vi "CloseTrig.vi"(8 "error in (no error)":errorcluster, 10 "TrigName":string, 11 "PXI_MultiTrig in":refnum<class "PXI_MultiTrig.lvclass">) -> (0 "error out":errorcluster, 3 "PXI_MultiTrig out":refnum<class "PXI_MultiTrig.lvclass">)   [LabVIEW 2018, in "SyncPlugins.lvlib" / "PXI_MultiTrig.lvclass"]
uses:
  PXI_MultiTrig.lvclass
  PXI_MultiTrig.lvclass/PXI_MultiTrig.ctl
  Accessors/Write TimingSession.vi
  Accessors/Write Triggers.vi
  Accessors/Read TimingSession.vi
  Accessors/Read RefClkSession.vi
  Accessors/Read Triggers.vi
  <vilib>/Utility/error.llb/Error Cluster From Error Code.vi
  <vilib>/ErrorRing/Error Ring.xnode
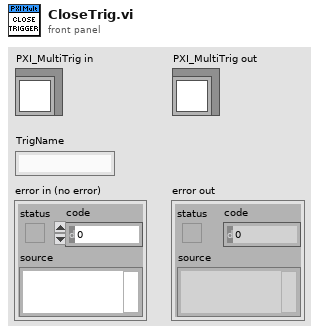
[diagram p1: front panel]
types:
  T1 = typedef "SyncPlugins.lvlib/PXI_MultiTrig.lvclass/clTrigger.ctl" = cluster{"Name":string, "DestTerm":string, "SrcTerm":string, "SyncClk":string, "Edge":i32, "Invert?":i32, "Initiated":bool, "Type":string, "TrigTime":bool}
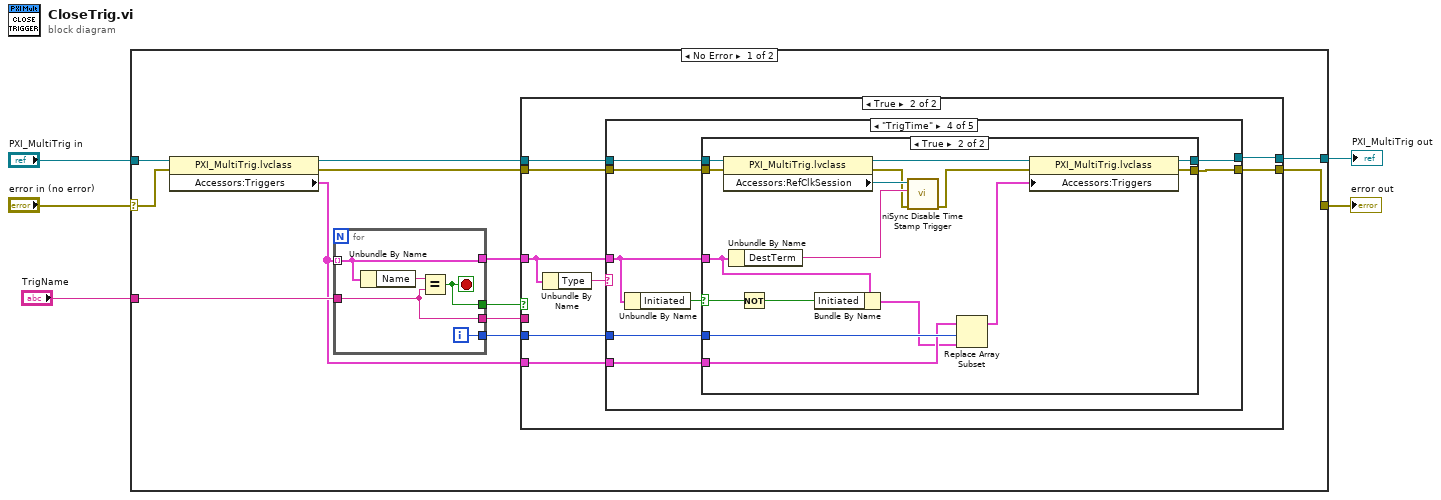
[diagram p0: block diagram]
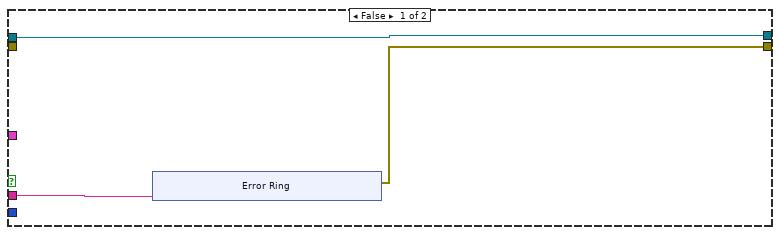
[diagram p2: hidden frame]
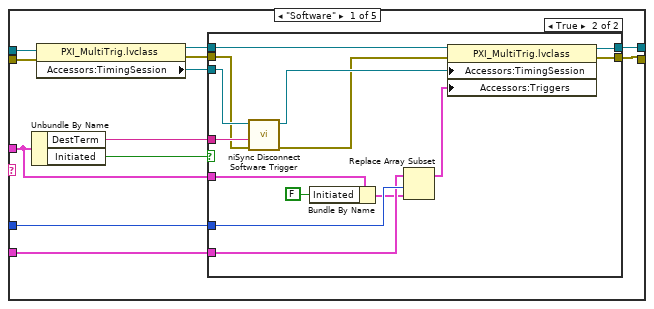
[diagram p3: hidden frame]
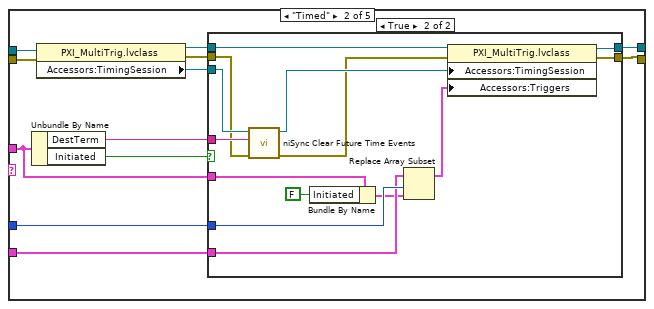
[diagram p5: hidden frame]
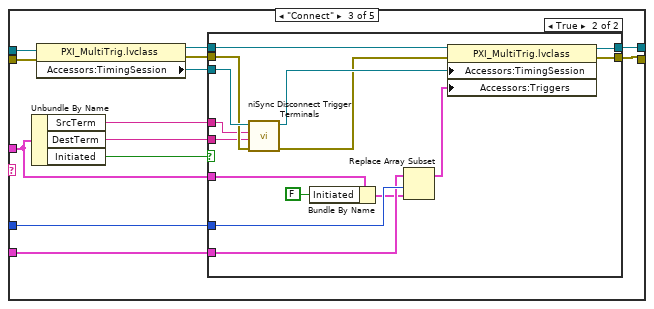
[diagram p7: hidden frame]
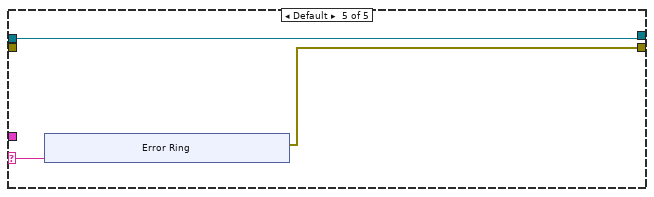
[diagram p10: hidden frame]
diagram:
  n1 = case shown="No Error" "error in (no error)" {
    selector: "error in (no error)" -> [w16 w163]
    tunnel: "PXI_MultiTrig in" -> [w17 w164]
    tunnel: "TrigName" -> [w15 _]
    tunnel: [w8 w164] -> w2
    tunnel: [w7 w163] -> w1
    frame No Error {
      n2 = property class="PXI_MultiTrig.lvclass"(reference=w17, error in=w16) -> (reference out=w12:refnum<class "PXI_MultiTrig.lvclass">, error out=w13:errorcluster, "Accessors:Triggers"=w6:T1[])
      n3 = for {
        tunnel: w6 -> [w161] mode=indexing
        tunnel: w15 -> [w159]
        tunnel: [w161] -> w11
        tunnel: [w160] -> w14
        tunnel: [w159] -> w10
        tunnel: [w158] -> w9
        i -> [w158]
        stop <- w160 stop-if-true
        n4 = Unbundle By Name(w161) -> ("Name"=w162:string)
        n5 = Equal?(x=w162, y=w159) -> (x = y?=w160:bool)
      }
      n6 = case shown="True" w14 {
        tunnel: w13 -> [_ w32]
        tunnel: w12 -> [w19 w33]
        tunnel: w11 -> [_ w31]
        tunnel: w10 -> [w20 _]
        tunnel: w9 -> [_ w28]
        tunnel: [w19 w30] -> w8
        tunnel: [w18 w34] -> w7
        tunnel: w6 -> [_ w29]
        frame False {
          n7 = xnode "Error Ring"("parameter 0"=w20) -> ("error out"=w18:errorcluster)
        }
        frame True {
          n8 = Unbundle By Name(w31) -> ("Type"=w35:string)
          n9 = case shown="\"TrigTime\"" w35 {
            selector: w35 -> [_ _ _ _ w150]
            tunnel: [w39 w67 w96 w124 w149] -> w34
            tunnel: w33 -> [w47 w75 w104 w126 w148]
            tunnel: w32 -> [w46 w74 w103 w127 _]
            tunnel: w31 -> [w37 w65 w94 w128 _]
            tunnel: [w40 w68 w97 w125 w148] -> w30
            tunnel: w29 -> [w38 w66 w95 w123 _]
            tunnel: w28 -> [w36 w64 w93 w122 _]
            frame "Software" {
              n10 = Unbundle By Name(w37) -> ("DestTerm"=w41:string, "Initiated"=w42:bool)
              n11 = property class="PXI_MultiTrig.lvclass"(reference=w47, error in=w46) -> (reference out=w45:refnum<class "PXI_MultiTrig.lvclass">, error out=w44:errorcluster, "Accessors:TimingSession"=w43:refnum<k15>)
              n12 = case shown="True" w42 {
                tunnel: w45 -> [w49 w53]
                tunnel: w44 -> [w48 w61]
                tunnel: w43 -> [_ w62]
                tunnel: w41 -> [_ w63]
                tunnel: [w49 w54] -> w40
                tunnel: [w48 w55] -> w39
                tunnel: w38 -> [_ w57]
                tunnel: w37 -> [_ w59]
                tunnel: w36 -> [_ w58]
                frame False {
                }
                frame True {
                  n13 = call <instrlib>:"niSync Disconnect Software Trigger.vi"("error in (no error)"=w61, "destination terminal"=w63, "instrument handle"=w62) -> ("error out"=w50:errorcluster, "instrument handle out"=w51:refnum<k15>)  [unwired: 7 in]
                  n14 = Bundle By Name(cluster=w59, "Initiated"=FALSE) -> (w56:T1)
                  n15 = Replace Array Subset(array=w57, new element=w56, index=w58) -> (w52:T1[])
                  n16 = property class="PXI_MultiTrig.lvclass"(reference=w53, error in=w50, "Accessors:TimingSession"=w51, "Accessors:Triggers"=w52) -> (reference out=w54:refnum<class "PXI_MultiTrig.lvclass">, error out=w55:errorcluster)
                }
              }
            }
            frame "Timed" {
              n17 = Unbundle By Name(w65) -> ("DestTerm"=w69:string, "Initiated"=w70:bool)
              n18 = property class="PXI_MultiTrig.lvclass"(reference=w75, error in=w74) -> (reference out=w73:refnum<class "PXI_MultiTrig.lvclass">, error out=w72:errorcluster, "Accessors:TimingSession"=w71:refnum<k15>)
              n19 = case shown="True" w70 {
                tunnel: w73 -> [w77 w81]
                tunnel: w72 -> [w76 w89]
                tunnel: w71 -> [_ w90]
                tunnel: w69 -> [_ w91]
                tunnel: [w77 w82] -> w68
                tunnel: [w76 w83] -> w67
                tunnel: w66 -> [_ w85]
                tunnel: w65 -> [_ w87]
                tunnel: w64 -> [_ w86]
                frame False {
                }
                frame True {
                  n20 = call <instrlib>:"niSync Clear Future Time Events.vi"("error in (no error)"=w89, "terminal"=w91, "instrument handle"=w90) -> ("error out"=w78:errorcluster, "instrument handle out"=w79:refnum<k15>)  [unwired: 6 in]
                  n21 = Bundle By Name(cluster=w87, "Initiated"=FALSE) -> (w84:T1)
                  n22 = Replace Array Subset(array=w85, new element=w84, index=w86) -> (w80:T1[])
                  n23 = property class="PXI_MultiTrig.lvclass"(reference=w81, error in=w78, "Accessors:TimingSession"=w79, "Accessors:Triggers"=w80) -> (reference out=w82:refnum<class "PXI_MultiTrig.lvclass">, error out=w83:errorcluster)
                }
              }
            }
            frame "Connect" {
              n24 = Unbundle By Name(w94) -> ("SrcTerm"=w92:string, "DestTerm"=w98:string, "Initiated"=w99:bool)
              n25 = property class="PXI_MultiTrig.lvclass"(reference=w104, error in=w103) -> (reference out=w102:refnum<class "PXI_MultiTrig.lvclass">, error out=w101:errorcluster, "Accessors:TimingSession"=w100:refnum<k15>)
              n26 = case shown="True" w99 {
                tunnel: w102 -> [w106 w112]
                tunnel: w101 -> [w105 w120]
                tunnel: w100 -> [_ w121]
                tunnel: w98 -> [_ w108]
                tunnel: [w106 w113] -> w97
                tunnel: [w105 w114] -> w96
                tunnel: w95 -> [_ w116]
                tunnel: w94 -> [_ w118]
                tunnel: w93 -> [_ w117]
                tunnel: w92 -> [_ w107]
                frame False {
                }
                frame True {
                  n27 = call <instrlib>:"niSync Disconnect Trigger Terminals.vi"("error in (no error)"=w120, "destination terminal"=w108, "source terminal"=w107, "instrument handle"=w121) -> ("error out"=w109:errorcluster, "instrument handle out"=w110:refnum<k15>)  [unwired: 6 in]
                  n28 = Bundle By Name(cluster=w118, "Initiated"=FALSE) -> (w115:T1)
                  n29 = Replace Array Subset(array=w116, new element=w115, index=w117) -> (w111:T1[])
                  n30 = property class="PXI_MultiTrig.lvclass"(reference=w112, error in=w109, "Accessors:TimingSession"=w110, "Accessors:Triggers"=w111) -> (reference out=w113:refnum<class "PXI_MultiTrig.lvclass">, error out=w114:errorcluster)
                }
              }
            }
            frame "TrigTime" {
              n31 = Unbundle By Name(w128) -> ("Initiated"=w129:bool)
              n32 = case shown="True" w129 {
                selector: w129 -> [_ w142]
                tunnel: w128 -> [_ w141]
                tunnel: w127 -> [w130 w146]
                tunnel: w126 -> [w131 w147]
                tunnel: [w131 w133] -> w125
                tunnel: [w130 w132] -> w124
                tunnel: w123 -> [_ w138]
                tunnel: w122 -> [_ w139]
                frame False {
                }
                frame True {
                  n33 = property class="PXI_MultiTrig.lvclass"(reference=w147, error in=w146) -> (reference out=w136:refnum<class "PXI_MultiTrig.lvclass">, error out=w143:errorcluster, "Accessors:RefClkSession"=w145:refnum<k15>)
                  n34 = Unbundle By Name(w141) -> ("DestTerm"=w144:string)
                  n35 = Not(x=w142) -> (.not. x?=w140:bool)
                  n36 = Bundle By Name(cluster=w141, "Initiated"=w140) -> (w137:T1)
                  n37 = call <instrlib>:"niSync Disable Time Stamp Trigger.vi"("error in (no error)"=w143, "terminal"=w144, "instrument handle"=w145) -> ("error out"=w135:errorcluster)  [unwired: 6 in, 1 out]
                  n38 = Replace Array Subset(array=w138, new element=w137, index=w139) -> (w134:T1[])
                  n39 = property class="PXI_MultiTrig.lvclass"(reference=w136, error in=w135, "Accessors:Triggers"=w134) -> (reference out=w133:refnum<class "PXI_MultiTrig.lvclass">, error out=w132:errorcluster)
                }
              }
            }
            frame Default {
              n40 = xnode "Error Ring"("parameter 0"=w150) -> ("error out"=w149:errorcluster)
            }
          }
        }
      }
    }
    frame Error {
    }
  }
  "error out" <- w1
  "PXI_MultiTrig out" <- w2
